vi "[RE Python] Part 1.vi"(8 "Error In":errorcluster, 11 "Fabric":i32[][](array[numeric])) -> (0 "Error Out":errorcluster, 3 "Sq in of Overlapping Claims":i32)   [LabVIEW 2019]
doc: "Given the Fabric from \"[RE Python] Build Fabric of Claims\", determine the number of spaces that have at least 2 claims (i.e. total area of overlapping claims)."
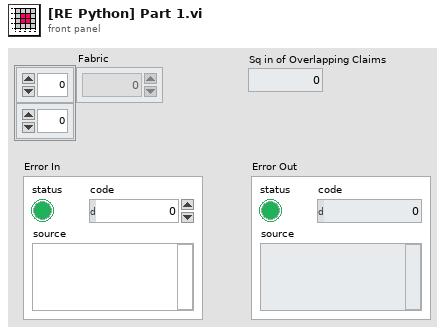
[diagram p1: front panel]
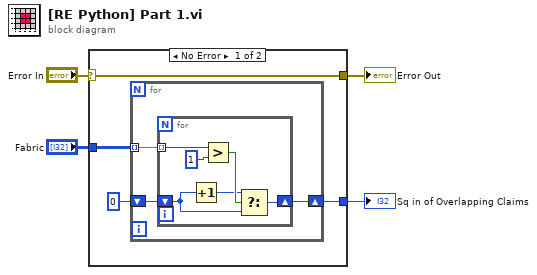
[diagram p0: block diagram]
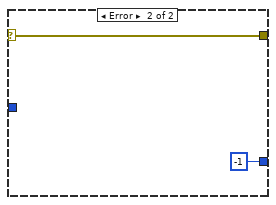
[diagram p2: hidden frame]
diagram:
  n1 = case shown="No Error" "Error In" {
    selector: "Error In" -> [w5 w19]
    tunnel: [w8 -1] -> w4
    tunnel: "Fabric" -> [w7 _]
    tunnel: [w5 w19] -> w1
    frame No Error {
      n2 = for {
        tunnel: w7 -> [w11] mode=indexing
        shift-right: [w10] -> w8
        shift-left: 0 -> [w9]
        n3 = for {
          tunnel: w11 -> [w17] mode=indexing
          shift-right: [w12] -> w10
          shift-left: w9 -> [w14]
          n4 = Increment(x=w14) -> (x+1=w13:i32)
          n5 = Greater?(x=w17, y=1) -> (0:w15:bool)
          n6 = Select(t=w13, s=w15, f=w14) -> (s? t:f=w12:i32)
        }
      }
    }
    frame Error {
    }
  }
  "Sq in of Overlapping Claims" <- w4
  "Error Out" <- w1
